vi "HEWH Data Cleanup.vi"(6 "60 Second Before Start":dbl, 8 "error in (no error)":errorcluster, 9 "Start Index":i32, 10 "Elapsed Time (sec)":dbl[](array[numeric]), 11 "Software Elapsed Time (sec)":dbl[](array[numeric])) -> (0 "error out":errorcluster, 3 "Search Element":dbl)   [LabVIEW 2020]
panel:
  out "End Index":i32
  out "Software Elapsed Time Clean":dbl[](array[numeric])
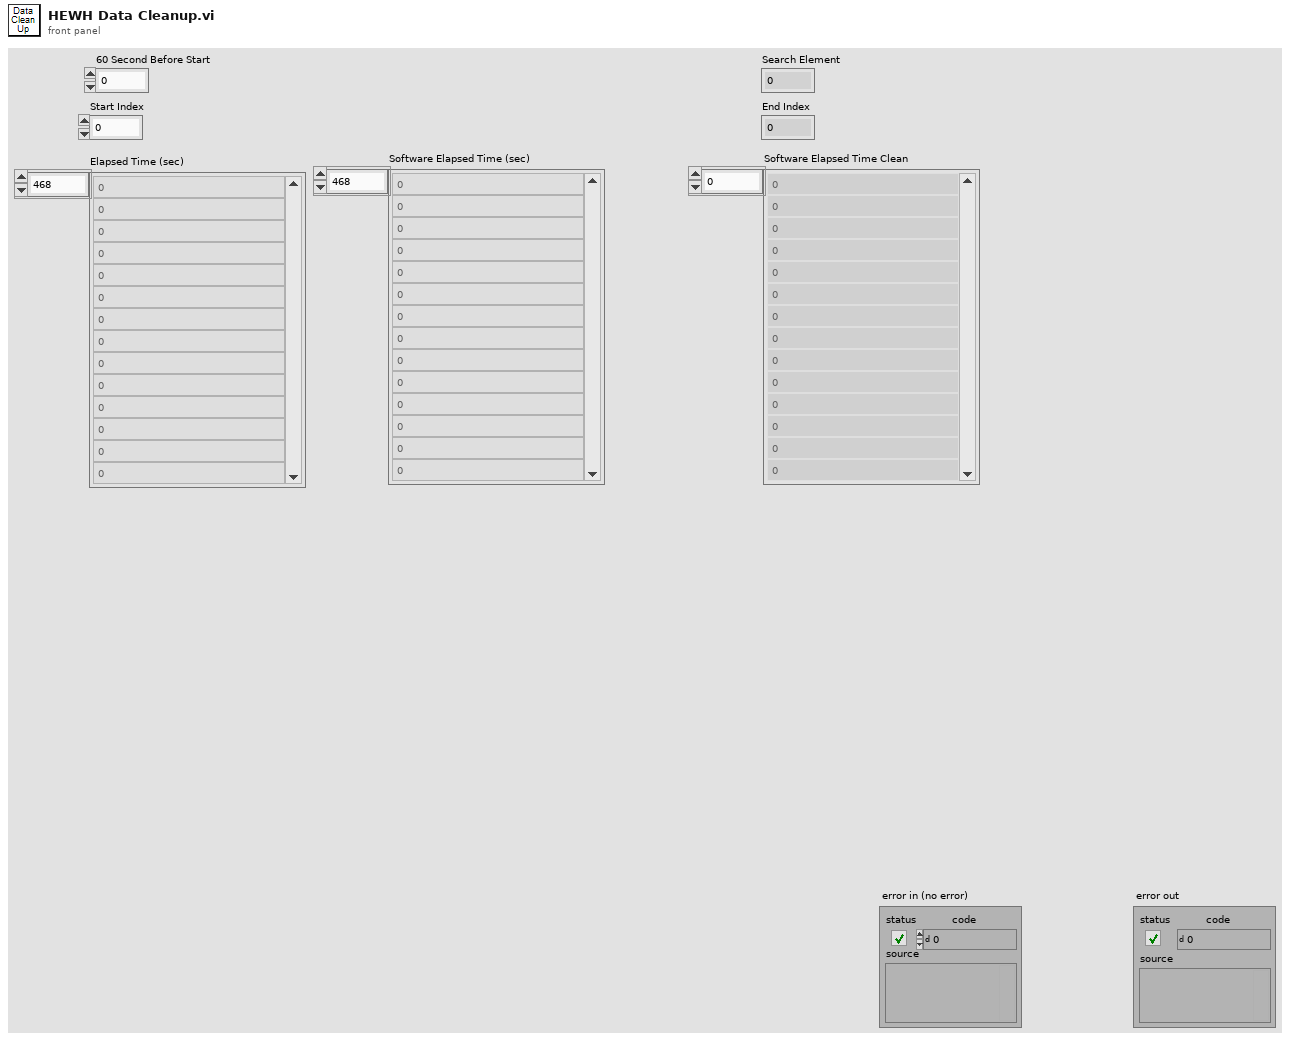
[diagram p1: front panel]
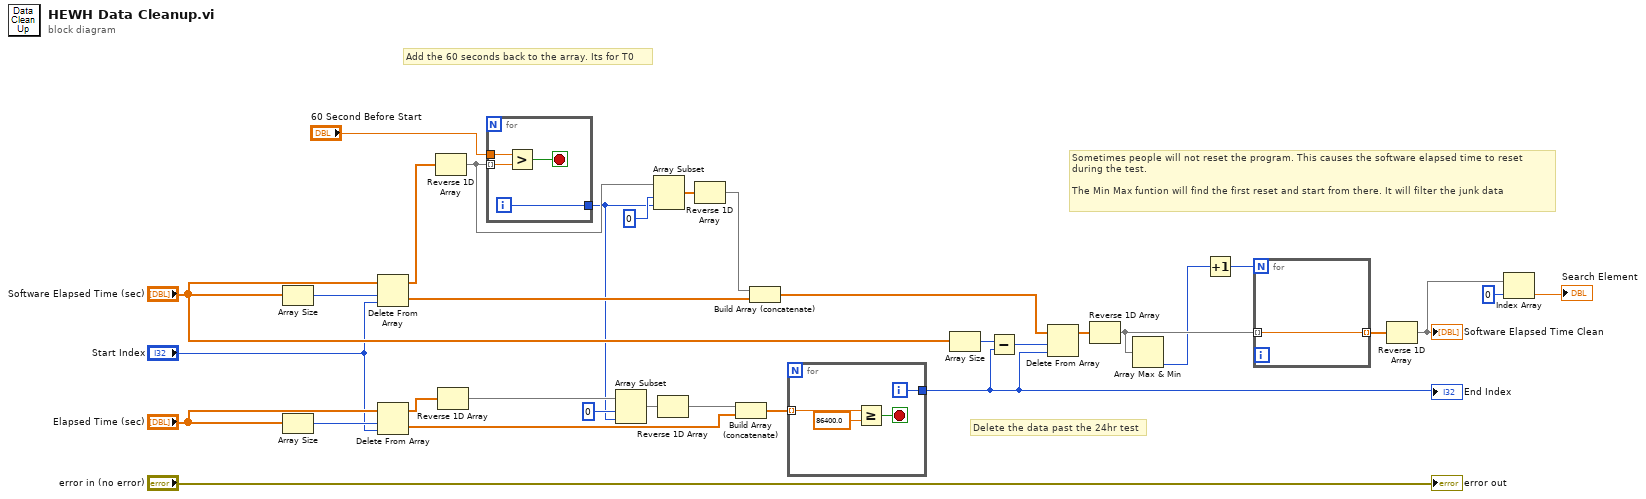
[diagram p0: block diagram]
diagram:
  # "Add the 60 seconds back to the array. Its for T0"
  # "Delete the data past the 24hr test"
  # "Sometimes people will not reset the program. This causes the software elapsed time to reset\nduring the test. \n\nThe Min Max funtion will find the first reset and start from there. It will filter the junk data"
  n1 = Array Size(array="Software Elapsed Time (sec)") -> (size(s)=w23:i32)
  n2 = Array Size(array="Elapsed Time (sec)") -> (size(s)=w21:i32)
  n3 = Delete From Array(array="Software Elapsed Time (sec)", length=w23, index="Start Index") -> (deleted portion=w14:dbl[], array with subset deleted=w19:dbl[])
  n4 = Delete From Array(array="Elapsed Time (sec)", length=w21, index="Start Index") -> (deleted portion=w6:dbl[], array with subset deleted=w12:dbl[])
  n5 = Reverse 1D Array(array=w19) -> (reversed array=w17:dbl[])
  n6 = Reverse 1D Array(array=w12) -> (reversed array=w9:dbl[])
  n7 = for {
    tunnel: w17 -> [w36] mode=indexing
    tunnel: "60 Second Before Start" -> [w37]
    tunnel: [w34] -> w8
    i -> [w34]
    stop <- w35 stop-if-true
    n8 = Greater?(x=w37, y=w36) -> (0:w35:bool)
  }
  n9 = Array Subset(array=w9, index=0, length=w8) -> (w11:dbl[])
  n10 = Array Subset(array=w17, index=0, length=w8) -> (w15:dbl[])
  n11 = Reverse 1D Array(array=w11) -> (reversed array=w7:dbl[])
  n12 = Reverse 1D Array(array=w15) -> (reversed array=w13:dbl[])
  n13 = Build Array (concatenate)(w7, w6) -> (w5:dbl[])
  n14 = Build Array (concatenate)(w13, w14) -> (w4:dbl[])
  n15 = for {
    tunnel: w5 -> [w41] mode=indexing
    tunnel: [w38] -> w28
    i -> [w38]
    stop <- w39 stop-if-true
    n16 = Greater Or Equal?(x=w41, y=86400.0) -> (x >= y?=w39:bool)
  }
  "End Index" <- w28
  n17 = Array Size(array="Software Elapsed Time (sec)") -> (size(s)=w29:i32)
  n18 = Subtract(x=w29, y=w28) -> (x-y=w27:i32)
  n19 = Delete From Array(array=w4, length=w27, index=w28) -> (array with subset deleted=w26:dbl[])  [unwired: 1 out]
  n20 = Reverse 1D Array(array=w26) -> (reversed array=w32:dbl[])
  n21 = Array Max & Min(array=w32) -> (min index (indices)=w31:i32)  [unwired: 3 out]
  n22 = Increment(x=w31) -> (x+1=w30:i32)
  n23 = for {
    N: w30 -> [_]
    tunnel: w32 -> [w42] mode=indexing
    tunnel: [w42] -> w25 mode=indexing
  }
  n24 = Reverse 1D Array(array=w25) -> (reversed array=w3:dbl[])
  "Software Elapsed Time Clean" <- w3
  n25 = Index Array(array=w3, index=0) -> (element=→"Search Element":dbl)
  "error out" <- "error in (no error)"
